vi "Can Stop.vi"(7 "Actor in":refnum<class "Actor.lvclass">, 8 "Error in":errorcluster, 10 "Msg Output":refnum<class "Msg Output.lvclass">) -> (0 "Error out":errorcluster, 2 "Stop":bool, 5 "Actor out":refnum<class "Actor.lvclass">)   [LabVIEW 2025, in "jettl.lvlib"]
uses:
  jettl.lvlib
  Actor/Actor.lvclass
  Msg Output/Msg Output.lvclass
  Stop Msg/Call.vi
  Stop Msg/Stop Msg.lvlib
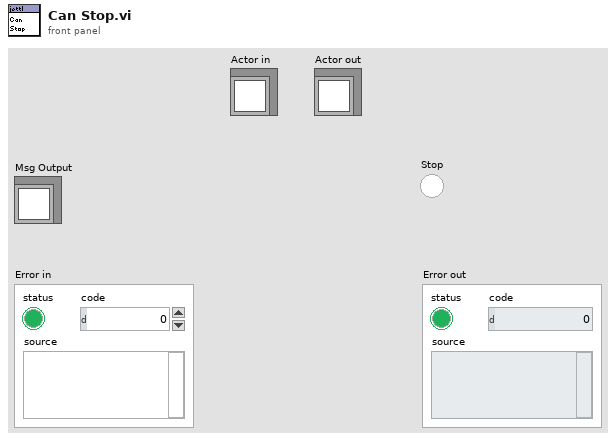
[diagram p1: front panel]
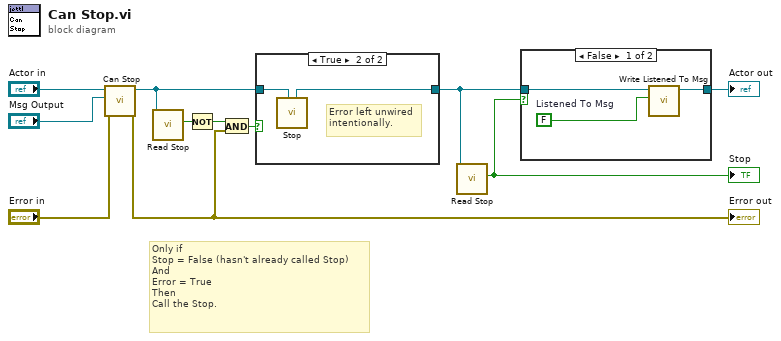
[diagram p0: block diagram]
diagram:
  # "Only if\nStop = False (hasn't already called Stop)\nAnd\nError = True\nThen\nCall the Stop."
  n1 = call-dynamic "Can Stop.vi"("Error in"="Error in", "Msg Output"="Msg Output", "Actor in"="Actor in") -> ("Error out"=w5:errorcluster, "Actor out"=w6:refnum<class "Actor.lvclass">)  [unwired: 7 in]
  "Error out" <- w5
  n2 = call-dynamic "Read Stop.vi"("Actor in"=w6) -> ("Stop"=w7:bool)  [unwired: 10 in]
  n3 = Not(x=w7) -> (.not. x?=w9:bool)
  n4 = And(x=w9, y=w5) -> (x .and. y?=w8:bool)
  n5 = case shown="True" w8 {
    tunnel: [w12 w13] -> w4
    tunnel: w6 -> [w12 w14]
    frame False {
    }
    frame True {
      # "Error left unwired intentionally."
      n6 = call-poly "Stop.vi"("Actor in"=w14) -> ("Actor out"=w13:refnum<class "Actor.lvclass">)  [unwired: 9 in, 1 out]
    }
  }
  n7 = call-dynamic "Read Stop.vi"("Actor in"=w4) -> ("Stop"=w2:bool)  [unwired: 10 in]
  "Stop" <- w2
  n8 = case shown="False" w2 {
    tunnel: w4 -> [w17 w18]
    tunnel: [w16 w18] -> w3
    frame False {
      w15 = FALSE  # Listened To Msg
      n9 = call-dynamic "Write Listened To Msg.vi"("Listened To Msg"=w15, "Actor in"=w17) -> ("Actor out"=w16:refnum<class "Actor.lvclass">)  [unwired: 9 in]
    }
    frame True {
    }
  }
  "Actor out" <- w3
